vi "Support_CheckLogComment.vi"(2 "log":T1[](array[typedef]) {"timestamp" format="%<%H:%M:%S%2u\n%Y/%m/%d>T"}, 3 "wanted comments":string[](array[string]), 5 "error in (no error)":errorcluster, 7 "start index":i32, 9 "length":i32=-1) -> (16 "Correct comments?":bool, 19 "error out":errorcluster)   [LabVIEW 2009]
doc: "Checks if wanted comments is same as logged call order."
uses:
  Support_LogType.ctl
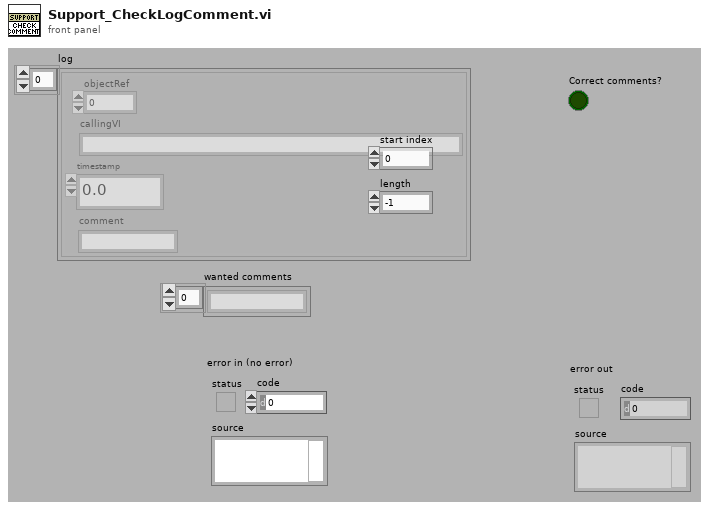
[diagram p1: front panel]
types:
  T1 = typedef "Support_LogType.ctl" = cluster{"objectRef":i32, "callingVI":string, "timestamp":dbl, "comment":string}
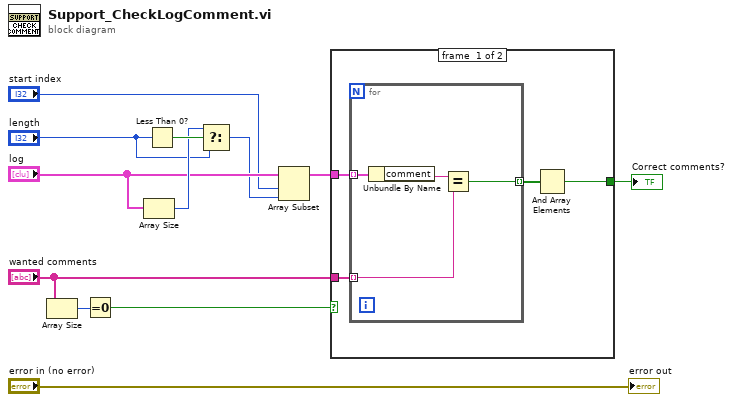
[diagram p0: block diagram]
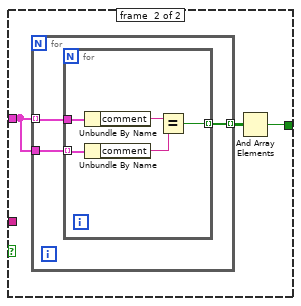
[diagram p2: hidden frame]
diagram:
  n1 = Array Size(array="wanted comments") -> (size(s)=w3:i32)
  n2 = Equal To 0?(x=w3) -> (x = 0?=w1:bool)
  n3 = Array Size(array="log") -> (size(s)=w9:i32)
  n4 = Less Than 0?(x="length") -> (x < 0?=w10:bool)
  n5 = Select(t=w9, s=w10, f="length") -> (s? t:f=w4:i32)
  n6 = Array Subset(array="log", index="start index", length=w4) -> (w7:T1[])
  n7 = case shown="True" w1 {
    tunnel: [w15 w22] -> w11
    tunnel: w7 -> [w14 w23]
    tunnel: "wanted comments" -> [w13 _]
    frame #0 {
      n8 = for {
        tunnel: w14 -> [w20] mode=indexing
        tunnel: w13 -> [w18] mode=indexing
        tunnel: [w17] -> w16 mode=indexing
        n9 = Unbundle By Name(w20) -> ("comment"=w19:string)
        n10 = Equal?(x=w19, y=w18) -> (x = y?=w17:bool)
      }
      n11 = And Array Elements(Boolean array=w16) -> (logical AND=w15:bool)
    }
    frame #1 {
      n12 = for {
        tunnel: w23 -> [w25] mode=indexing
        tunnel: w23 -> [w26]
        tunnel: [w24] -> w21 mode=indexing
        n13 = for {
          tunnel: w26 -> [w30] mode=indexing
          tunnel: w25 -> [w31]
          tunnel: [w27] -> w24 mode=indexing
          n14 = Unbundle By Name(w31) -> ("comment"=w29:string)
          n15 = Unbundle By Name(w30) -> ("comment"=w28:string)
          n16 = Equal?(x=w29, y=w28) -> (x = y?=w27:bool)
        }
      }
      n17 = And Array Elements(Boolean array=w21) -> (logical AND=w22:bool)
    }
  }
  "Correct comments?" <- w11
  "error out" <- "error in (no error)"
